vi "DAQ_thermometer_DAQ_Project.vi"() -> ()   [LabVIEW 2020]
uses:
  <vilib>/DAQmx/read.llb/DAQmx Read (Analog 2D DBL NChan NSamp).vi
  <vilib>/DAQmx/create/channels.llb/DAQmx Create Channel (AI-Temperature-Thermocouple).vi
  <vilib>/DAQmx/configure/timing.llb/DAQmx Timing (Sample Clock).vi
  <vilib>/DAQmx/miscellaneous.llb/DAQmx Fill In Error Info.vi
panel:
  out "Display Values":dbl[][](array[numeric])
  in  "file path (use dialog)":path
  out "Waveform Graph":dbl[][](graph)
  in  "number of samples per channel":i32=-1
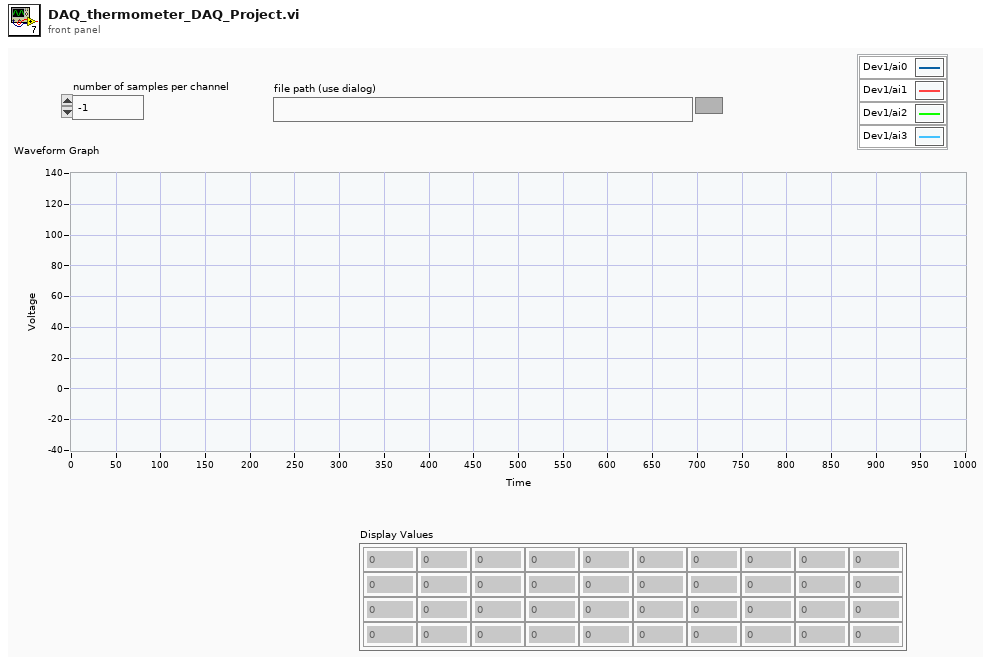
[diagram p1: front panel]
types:
  T1 = enum16{"open", "replace", "create", "open or create", "replace or create", "replace or create with confirmation"}
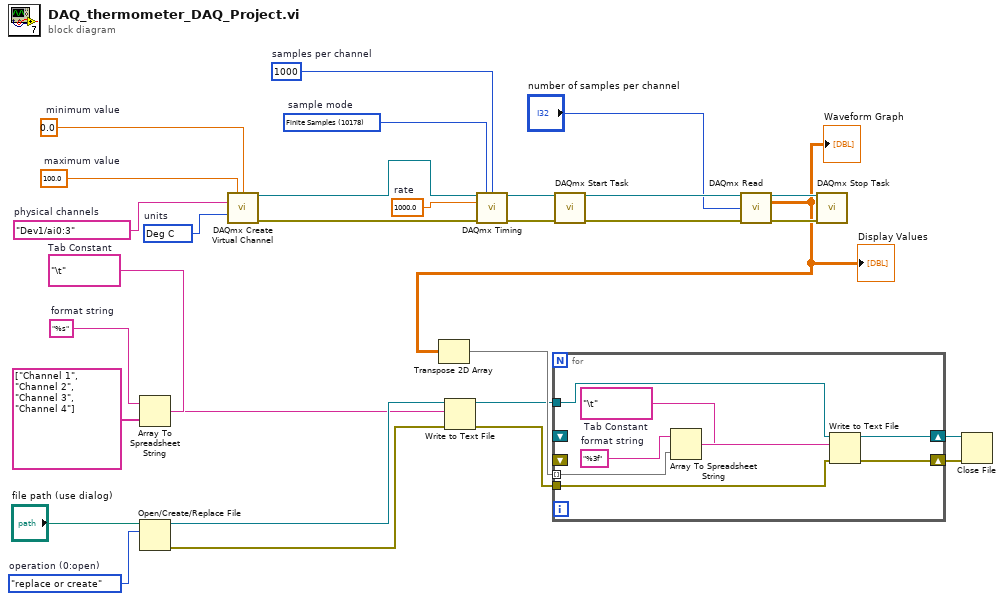
[diagram p0: block diagram]
diagram:
  w2 = "%s"  # format string
  w9 = "\t"  # Tab Constant
  w11 = T1."replace or create"  # operation (0:open)
  w16 = 10143 items=["Deg C"=10143, "Deg F"=10144, "Kelvins"=10325, "Deg R"=10145, "From Custom Scale"=10065]  # units
  w17 = 1000  # samples per channel
  w18 = 10178 items=["Finite Samples"=10178, "Continuous Samples"=10123, "Hardware Timed Single Point"=12522]  # sample mode
  w19 = 1000.0  # rate
  w20 = 0.0  # minimum value
  w21 = 100.0  # maximum value
  w22 = tag "Dev1/ai0:3"  # physical channels
  n1 = Array To Spreadsheet String(delimiter (Tab)=w9, array=string[] ["Channel 1", "Channel 2", "Channel 3", "Channel 4"], 3:w2) -> (spreadsheet string=w5:string)
  n2 = Open/Create/Replace File(file path (use dialog)="file path (use dialog)", operation (0:open)=w11) -> (refnum out=w14:refnum<file>, error out=w13:errorcluster)  [unwired: 4 in, 1 out]
  n3 = call-poly <vilib>:"DAQmx Create Virtual Channel.vi"("maximum value"=w21, "minimum value"=w20, "physical channels"=w22, "units"=w16) -> ("task out"=w30:refnum<k21>, "error out"=w29:errorcluster)  [unwired: 10 in]
  n4 = Write to Text File(file (use dialog)=w14, text=w5, error in=w13) -> (refnum out=w4:refnum<file>, error out=w3:errorcluster)  [unwired: 1 in, 1 out]
  n5 = call-poly <vilib>:"DAQmx Timing.vi"("task/channels in"=w30, "sample mode"=w18, "samples per channel"=w17, "rate"=w19, "error in"=w29) -> ("task out"=w28:refnum<k21>, "error out"=w27:errorcluster)  [unwired: 9 in]
  n6 = call <vilib>:"DAQmx Start Task.vi"("task/channels in"=w28, "error in"=w27) -> ("task out"=w26:refnum<k21>, "error out"=w25:errorcluster)  [unwired: 12 in]
  n7 = call-poly <vilib>:"DAQmx Read.vi"("task/channels in"=w26, "number of samples per channel"="number of samples per channel", "error in"=w25) -> ("task out"=w24:refnum<k21>, "data"=w1:dbl[][], "error out"=w23:errorcluster)  [unwired: 10 in]
  "Waveform Graph" <- w1
  "Display Values" <- w1
  n8 = Transpose 2D Array(2D array=w1) -> (transposed array=w6:dbl[][])
  n9 = for {
    shift-right: [w38] -> w8
    shift-left: _ -> [_]
    shift-right: [w37] -> w7
    shift-left: _ -> [_]
    tunnel: w6 -> [w34] mode=indexing
    tunnel: w4 -> [w33]
    tunnel: w3 -> [w32]
    w31 = "%3f"  # format string
    w35 = "\t"  # Tab Constant
    n10 = Array To Spreadsheet String(delimiter (Tab)=w35, array=w34, 3:w31) -> (spreadsheet string=w36:string)
    n11 = Write to Text File(file (use dialog)=w33, text=w36, error in=w32) -> (refnum out=w38:refnum<file>, error out=w37:errorcluster)  [unwired: 1 in, 1 out]
  }
  n12 = call <vilib>:"DAQmx Stop Task.vi"("task/channels in"=w24, "error in"=w23) -> ()  [unwired: 12 in, 2 out]
  n13 = Close File(refnum=w8, error in=w7) -> ()  [unwired: 2 out]
